vi "Global 4.vi"() -> ()   [LabVIEW 2018]
panel:
  out "Min":dbl(slide) scale=0.0..100.0
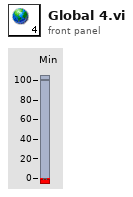
[diagram p1: front panel]
diagram:
